vi "read_from_file.vi"(11 "file (use dialog)":path) -> (3 "data":bool[](array[boolean]))   [LabVIEW 2013]
panel:
  in  "Boolean":bool
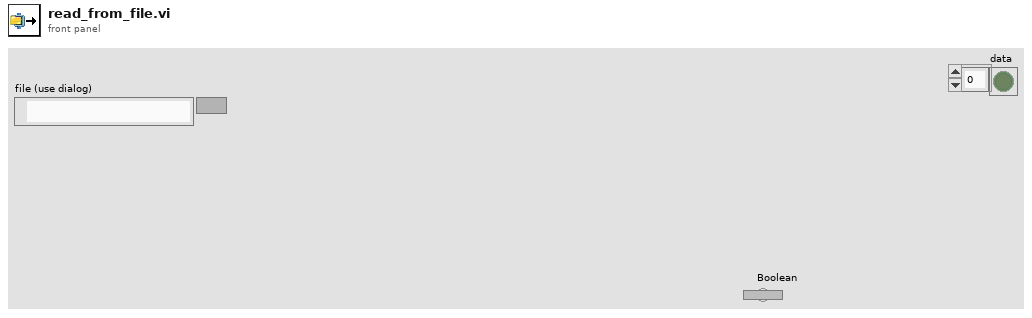
[diagram p1: front panel]
types:
  T1 = enum16{"open", "replace", "create", "open or create", "replace or create", "replace or create with confirmation"}
  T2 = enum16{"big-endian, network order", "native, host order", "little-endian"}
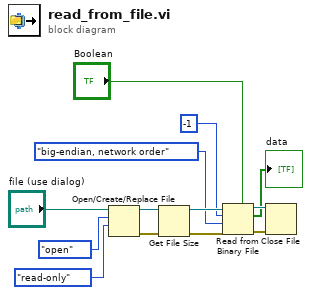
[diagram p0: block diagram]
diagram:
  n1 = Open/Create/Replace File(file path (use dialog)="file (use dialog)", operation (0:open)=T1."open", access (0:read/write)=enum16{"read/write", "read-only", "write-only"}."read-only") -> (refnum out=w12:refnum<file>, error out=w5:errorcluster)  [unwired: 3 in, 1 out]
  n2 = Get File Size(file=w12, error in=w5) -> (refnum out=w13:refnum<file>, 0:w4:errorcluster)  [unwired: 1 out]
  n3 = Read from Binary File(5:"Boolean", 8:w4, 9:T2."big-endian, network order" ("byte order (0:big-endian, network order)"), 10:-1 ("count (1)"), 11:w13) -> (0:w3:errorcluster, 2:→"data":bool[], 3:w6:refnum<file>)  [unwired: 1 in, 1 out]
  n4 = Close File(refnum=w6, error in=w3) -> ()  [unwired: 2 out]
